vi "View configurations.vi"(8 "error in (no error)":errorcluster) -> (0 "error out":errorcluster)   [LabVIEW 2012, in "ServiceManager.lvclass"]
uses:
  ServiceManager.lvclass
  <vilib>/Utility/miscctls.llb/LVPointTypeDef.ctl
  Murmex/LabVIEW/Murmex/Murmex/configuration_cluster.ctl
  <vilib>/Distrio/LabbitMQ/Connection/connection_parameters_cluster.ctl
  Murmex/LabVIEW/Murmex/Murmex/observers_cluster.ctl
  Murmex/LabVIEW/Murmex/Murmex/observer_cluster_2.ctl
  Murmex/LabVIEW/Murmex/Murmex/observe_mode_enum.ctl
  Murmex/LabVIEW/Murmex/Murmex/Queue type enum.ctl
  ServiceManager.lvclass/ServiceManager.ctl
  Murmex/LabVIEW/Murmex/Murmex/Murmex.lvclass
  <vilib>/Distrio/LabbitMQ/Connection/Connection.lvclass
panel:
  in  "button:refresh":bool
  in  "button:ok":bool
  in  "Tree":string(tree)
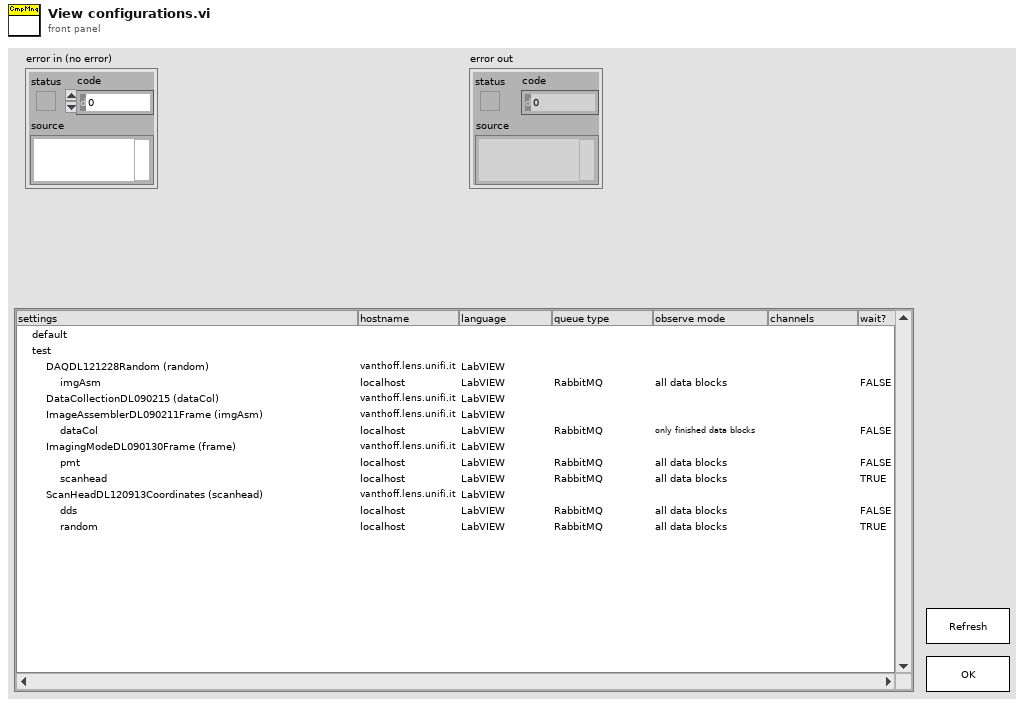
[diagram p1: front panel]
types:
  T1 = typedef "Murmex.lvlib/Murmex.lvclass/configuration_cluster.ctl" = cluster{"connection parameters":T2, "observers":T3, "mapping script":string, "window positions":cluster{"visibility":string, "left":i16, "top":i16}}
  T2 = typedef "Connection.lvclass/connection_parameters_cluster.ctl" = cluster{"host name":string, "port":i32, "user name":string, "password":string, "virtual host":string}
  T3 = typedef "Murmex.lvlib/Murmex.lvclass/observers_cluster.ctl" = cluster{"observer":T4[]}
  T4 = typedef "Murmex.lvlib/Murmex.lvclass/observer_cluster_2.ctl" = cluster{"ID":string, "observe mode":T5, "channels":string, "queue type":T6, "wait until done?":bool}
  T5 = typedef "Murmex.lvlib/Murmex.lvclass/observe_mode_enum.ctl" = enum16{"all data blocks", "only finished data blocks"}
  T6 = typedef "Murmex.lvlib/Murmex.lvclass/Queue type enum.ctl" = enum16{"RabbitMQ", "Network streaming queue"}
  T7 = typedef "LVPointTypeDef.ctl" = cluster{"Horizontal":i16, "Vertical":i16}
  T8 = typedef "ServiceManager.lvclass/settings_cluster.ctl" = cluster{"components":T9[], "compile projects":bool}
  T9 = typedef "Murmex.lvlib/Murmex.lvclass/component_specification_cluster.ctl" = cluster{"name":string, "language":string, "host name":string, "id":string}
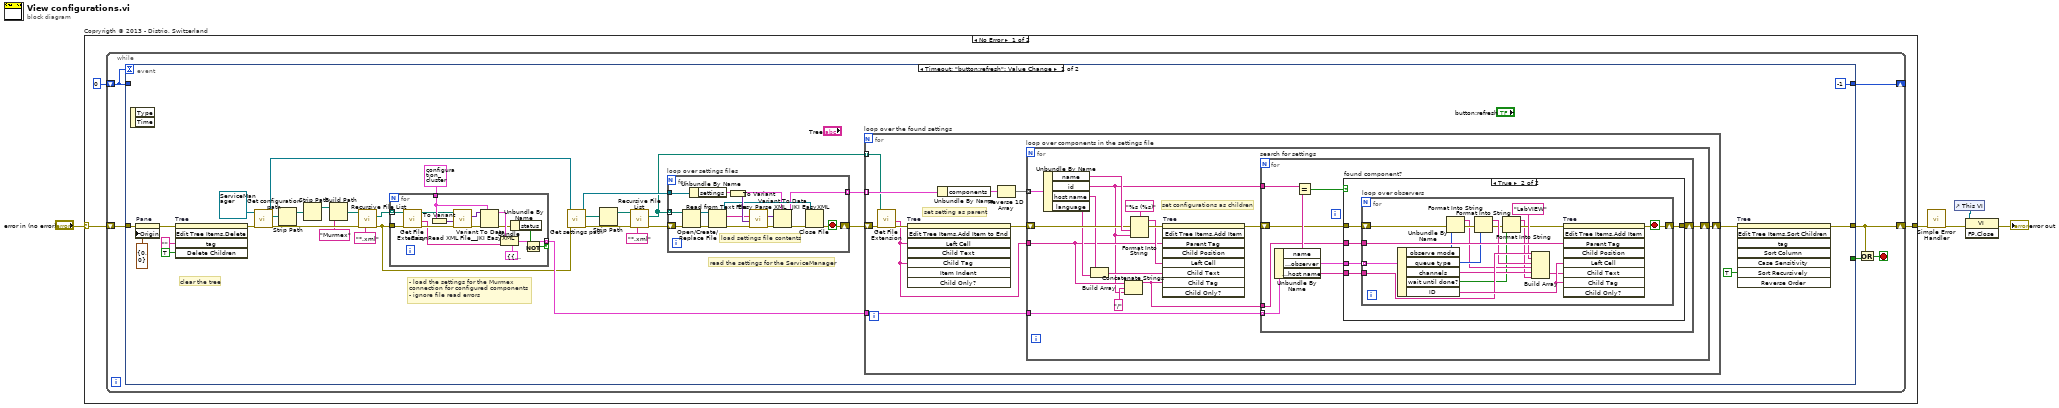
[diagram p0: block diagram]
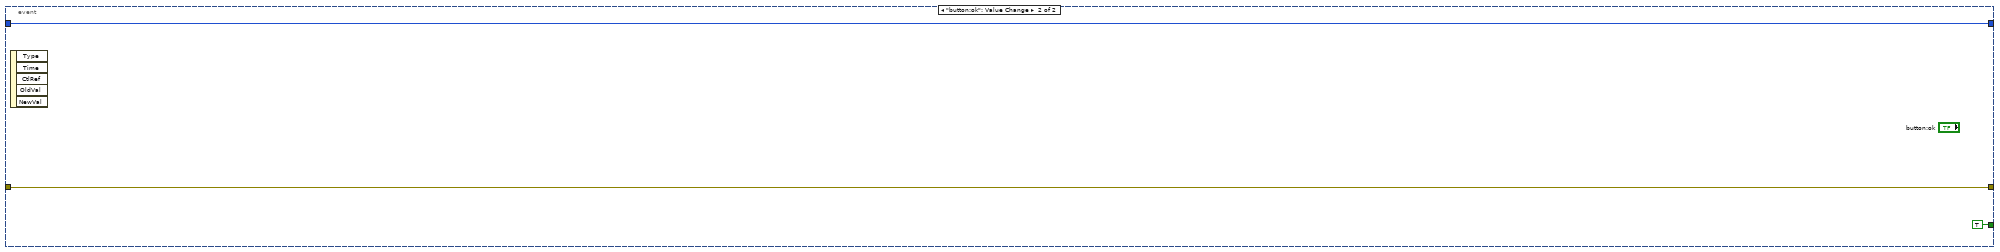
[diagram p3: hidden frame]
diagram:
  n1 = case "Copryrigth © 2013 - Distrio, Switzerland" shown="No Error" "error in (no error)" {
    selector: "error in (no error)" -> [w7 w139]
    tunnel: [w8 w139] -> w4
    frame No Error {
      n2 = while {
        shift-right: [w13] -> w8
        shift-left: w7 -> [w14]
        shift-right: [w9] -> _
        shift-left: 0 -> [w10]
        stop <- w11 stop-if-true
        n3 = event shown="[0] Timeout;  \"button:refresh\": Value Change" {
          selector: _ -> [_ _]
          dyn-events: _ -> [_ _]
          timeout: w10 -> [_ _]
          tunnel: w14 -> [w35 w136]
          tunnel: [w21 w136] -> w13
          tunnel: [_ TRUE] -> w12
          tunnel: w10 -> [_ w138]
          tunnel: [-1 w138] -> w9
          event Timeout; "button:refresh": Value Change {
            # "read the settings for the ServiceManager"
            # "- load the settings for the Murmex\nconnection for configured components\n- ignore file read errors"
            # "clear the tree"
            n4 = event-data() -> ()  [unwired: 1 in, 2 out]
            n5 = property on="Pane" class="Pane"(error in=w35, "Origin"=T7 {"Horizontal"=0, "Vertical"=0}) -> (error out=w34:errorcluster)  [unwired: 1 in, 1 out]
            n6 = invoke on="Tree" class="Tree (strict)" method="Edit Tree Items.Delete"(error in=w34, "tag"="" ("Tag"), "Delete Children"=TRUE ("Delete Children?")) -> (error out=w36:errorcluster)  [unwired: 2 in, 4 out]
            n7 = call "Get configuration path.vi"("error in (no error)"=w36, "Murmex in"=refnum<class "ServiceManager.lvclass"> refnum ("ServiceManager in")) -> ("error out"=w33:errorcluster, "configuration path"=w31:path, "Murmex out"=w29:refnum<class "ServiceManager.lvclass">)  [unwired: 7 in]
            n8 = Strip Path(path=w31) -> (stripped path=w25:path)  [unwired: 1 out]
            n9 = Strip Path(path=w25) -> (stripped path=w27:path)  [unwired: 1 out]
            n10 = Build Path(base path=w27, name or relative path="Murmex") -> (appended path=w24:path)
            n11 = call <vilib>:"Recursive File List.vi"("pattern"="*.xml", "error in (no error)"=w33, "Folder Path"=w24) -> ("error out"=w17:errorcluster, "All Files in Dir"=w30:path[])  [unwired: 4 in, 3 out]
            n12 = for {
              tunnel: w30 -> [w55] mode=indexing
              tunnel: T1 {"connection parameters"={"host name"="localhost", "port"=5672, "user name"="guest", "password"="guest", "virtual host"="/"}, "observers"={"observer"=[]}, "mapping script"="", "window positions"={"visibility"="", "left"=0, "top"=0}} ("configuration") -> [w58]
              tunnel: [w53] -> w23 mode=indexing if=w47
              tunnel: w17 -> [w57]
              n13 = call <vilib>:"Get File Extension.vi"("error in (no error)"=w57, "file"=w55) -> ("error out"=w56:errorcluster, "filename without extension"=w50:string, "dup file"=w54:path)  [unwired: 6 in, 1 out]
              n14 = To Variant(anything=w58) -> (Variant=w61:variant)
              n15 = call <vilib>:"Easy Read XML File__JKI EasyXML.vi"("error in (no error)"=w56, "LabVIEW Data (Type)"=w61, "XML File Path"=w54) -> ("error out"=w59:errorcluster, "LabVIEW Data"=w60:variant)  [unwired: 6 in, 1 out]
              n16 = Variant To Data(error in=w59, type=w58, Variant=w60) -> (data=w51:T1, error out=w49:errorcluster)
              n17 = Bundle(cluster=cluster{"configuration":T1, "name":string} {"configuration"={"connection parameters"={"host name"="", "port"=0, "user name"="", "password"="", "virtual host"=""}, "observers"={"observer"=[]}, "mapping script"="", "window positions"={"visibility"="", "left"=0, "top"=0}}, "name"=""}, "configuration"=w51, "name"=w50) -> (w53:cluster{"configuration":T1, "name":string})
              n18 = Unbundle By Name(w49) -> ("status"=w48:bool)
              n19 = Not(x=w48) -> (.not. x?=w47:bool)
            }
            n20 = call-dynamic "Get settings path.vi"("error in (no error)"=w17, "Murmex in"=w29) -> ("error out"=w46:errorcluster, "settings path"=w16:path, "Murmex out"=w43:refnum<class "ServiceManager.lvclass">)  [unwired: 7 in]
            n21 = Strip Path(path=w16) -> (stripped path=w15:path)  [unwired: 1 out]
            n22 = call <vilib>:"Recursive File List.vi"("pattern"="*.xml", "error in (no error)"=w46, "Folder Path"=w15) -> ("error out"=w44:errorcluster, "All Files in Dir"=w41:path[])  [unwired: 4 in, 3 out]
            n23 = for "loop over settings files" {
              tunnel: w41 -> [w135] mode=indexing
              shift-right: [w121] -> w40
              shift-left: w44 -> [w134]
              tunnel: w43 -> [w133]
              tunnel: [w122] -> w42 mode=indexing
              stop <- w121 stop-if-true
              # "load settings file contents"
              n24 = Open/Create/Replace File(file path (use dialog)=w135, error in=w134) -> (refnum out=w128:refnum<file>, error out=w129:errorcluster)  [unwired: 4 in, 1 out]
              n25 = Unbundle By Name(w133) -> ("settings"=w123:T8)
              n26 = Read from Text File(file (use dialog)=w128, error in=w129) -> (refnum out=w125:refnum<file>, text=w127:string, error out=w126:errorcluster)  [unwired: 2 in, 1 out]
              n27 = To Variant(anything=w123) -> (Variant=w131:variant)
              n28 = call <vilib>:"Easy Parse XML__JKI EasyXML.vi"("error in (no error)"=w126, "LabVIEW Data (Type)"=w131, "XML String"=w127) -> ("error out"=w130:errorcluster, "LabVIEW Data"=w132:variant)  [unwired: 7 in]
              n29 = Variant To Data(error in=w130, type=w123, Variant=w132) -> (data=w122:T8, error out=w124:errorcluster)
              n30 = Close File(refnum=w125, error in=w124) -> (error out=w121:errorcluster)  [unwired: 1 out]
            }
            n31 = for "loop over the found settings" {
              tunnel: w42 -> [w71] mode=indexing
              tunnel: w41 -> [w69] mode=indexing
              shift-right: [w65] -> w22
              shift-left: w40 -> [w70]
              tunnel: w23 -> [w62]
              # "set setting as parent"
              n32 = call <vilib>:"Get File Extension.vi"("error in (no error)"=w70, "file"=w69) -> ("error out"=w68:errorcluster, "filename without extension"=w63:string)  [unwired: 6 in, 2 out]
              n33 = invoke on="Tree" class="Tree (strict)" method="Edit Tree Items.Add Item to End"(error in=w68, "Left Cell"=w63, "Child Tag"=w63) -> (error out=w66:errorcluster)  [unwired: 5 in, 7 out]
              n34 = Unbundle By Name(w71) -> ("components"=w67:T9[])
              n35 = Reverse 1D Array(array=w67) -> (reversed array=w64:T9[])
              n36 = for "loop over components in the settings file" {
                tunnel: w64 -> [w87] mode=indexing
                tunnel: w63 -> [w75]
                shift-right: [w76] -> w65
                shift-left: w66 -> [w85]
                tunnel: w62 -> [w78]
                # "set configurations as children"
                n37 = Unbundle By Name(w87) -> ("name"=w86:string, "id"=w73:string, "host name"=w81:string, "language"=w80:string)
                n38 = Build Array(w81, w80) -> (w79:string[])
                n39 = Concatenate Strings(w75, "/" ("string"), w73) -> (w72:string)
                n40 = Format Into String(format string="%s (%s)", error in=w85, w86, w73) -> (resulting string=w82:string, error out=w84:errorcluster)  [unwired: 1 in]
                n41 = invoke on="Tree" class="Tree (strict)" method="Edit Tree Items.Add Item"(error in=w84, "Parent Tag"=w75, "Left Cell"=w82, "Child Text"=w79, "Child Tag"=w72) -> (error out=w77:errorcluster)  [unwired: 4 in, 8 out]
                n42 = for "search for settings" {
                  tunnel: w78 -> [w96] mode=indexing
                  tunnel: w73 -> [w88]
                  shift-right: [w91] -> w76
                  shift-left: w77 -> [w92]
                  tunnel: w72 -> [w89]
                  n43 = Unbundle By Name(w96) -> ("name"=w95:string, "configuration.observers.observer"=w93:T4[], "configuration.connection parameters.host name"=w90:string)
                  n44 = Equal?(x=w88, y=w95) -> (x = y?=w94:bool)
                  n45 = case "found component?" shown="True" w94 {
                    tunnel: w93 -> [_ w102]
                    tunnel: w92 -> [w97 w101]
                    tunnel: w89 -> [_ w100]
                    tunnel: [w97 w99] -> w91
                    tunnel: w90 -> [_ w98]
                    frame False {
                    }
                    frame True {
                      n46 = for "loop over observers" {
                        tunnel: w102 -> [w120] mode=indexing
                        tunnel: w100 -> [w118]
                        shift-right: [w107] -> w99
                        shift-left: w101 -> [w117]
                        tunnel: w98 -> [w116]
                        stop <- w107 stop-if-true
                        n47 = Unbundle By Name(w120) -> ("observe mode"=w115:T5, "queue type"=w113:T6, "channels"=w112:string, "wait until done?"=w104:bool, "ID"=w119:string)
                        n48 = Format Into String(error in=w117, w115) -> (resulting string=w110:string, error out=w114:errorcluster)  [unwired: 2 in]
                        n49 = Format Into String(error in=w114, w113) -> (resulting string=w109:string, error out=w106:errorcluster)  [unwired: 2 in]
                        n50 = Format Into String(error in=w106, w104) -> (resulting string=w103:string, error out=w105:errorcluster)  [unwired: 2 in]
                        n51 = Build Array(w116, "LabVIEW" ("element"), w109, w110, w112, w103) -> (w111:string[])
                        n52 = invoke on="Tree" class="Tree (strict)" method="Edit Tree Items.Add Item"(error in=w105, "Parent Tag"=w118, "Left Cell"=w119, "Child Text"=w111, "Child Tag"=w119) -> (error out=w107:errorcluster)  [unwired: 4 in, 8 out]
                      }
                    }
                  }
                }
              }
            }
            n53 = invoke on="Tree" class="Tree (strict)" method="Edit Tree Items.Sort Children"(error in=w22, "Sort Recursively"=TRUE ("Sort Recursively?")) -> (error out=w21:errorcluster)  [unwired: 6 in, 7 out]
          }
          event "button:ok": Value Change {
            n54 = event-data() -> ()  [unwired: 1 in, 5 out]
          }
        }
        n55 = Or(x=w13, y=w12) -> (x .or. y?=w11:bool)
      }
    }
    frame Error {
    }
  }
  n56 = call <vilib>:"Simple Error Handler.vi"("error in (no error)"=w4) -> ("error out"=w2:errorcluster)  [unwired: 4 in, 4 out]
  n57 = control-ref of="This VI"() -> (w3:refnum<vi>)
  n58 = invoke class="VI" method="FP.Close"(reference=w3, error in=w2) -> (error out=→"error out":errorcluster)  [unwired: 1 in, 2 out]
